vi "Config Type.vi"(11 "SeqLoaded Condition in":refnum<class "SeqLoaded Condition.lvclass">) -> (2 "Condition Config":refnum<class "Condition Config.lvclass">)   [LabVIEW 2020, in "VolatusSeq.lvlib" / "SeqLoaded Condition.lvclass"]
uses:
  SeqLoaded Condition.lvclass
  SeqLoaded Condition.lvclass/SeqLoaded Condition.ctl
  VolatusSeqConfig/SeqLoaded Condition Config/SeqLoaded Condition Config.lvclass
  C:/dev/lv20CE/relink/lv-volatus/VolatusSeqConfig/Condition Config/Condition Config.lvclass
  C:/dev/lv20CE/relink/lv-volatus/VolatusSeqConfig/SeqLoaded Condition Config/SeqLoaded Condition Config.lvclass
  VolatusSeqConfig/Condition Config/Condition Config.lvclass
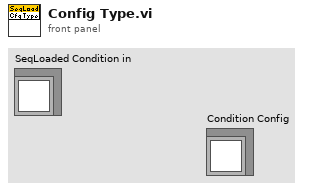
[diagram p1: front panel]
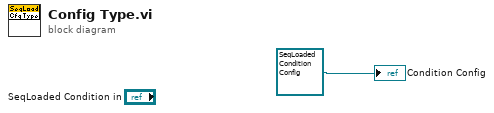
[diagram p0: block diagram]
diagram:
  "Condition Config" <- refnum<class "SeqLoaded Condition Config.lvclass"> refnum ("VolatusSeqConfig.lvlib:SeqLoaded Condition Config.lvclass")
